vi "Disabled.vi"(7 "Robot Mode":T3, 10 "Match Info":T2={"Autonomous Elapsed Seconds"=0.0, "TeleOp Elapsed Seconds"=0.0, "Disabled Elapsed Seconds"=0.0, "Visited Autonomous"=FALSE, "Visited TeleOp"=FALSE, "Visited Disabled"=FALSE, "Autonomous Settings"={"Autonomous Style"=enum."Independent", "VI Refnum"=refnum}}, 11 "Call Context":T4) -> ()   [LabVIEW 2016]
doc: "This VI is called each time a disabled packet is received from the DS. It is often used to prepare for the next robot mode, to calibrate sensors, etc."
uses:
  <vilib>/Rock Robotics/WPI/DriverStation/WPI_DriverStationDerivedRobotMode.ctl
  <vilib>/Rock Robotics/WPI/DriverStation/WPI_DriverStationRobotMode2.ctl
  <vilib>/Rock Robotics/WPI/DriverStation/WPI_DriverStationMatch Info.ctl
  <vilib>/Rock Robotics/WPI/ThirdParty/CanMotor/TalonSRX/WPI_CANTalonSRX_GlobalStatus.ctl
  <vilib>/Rock Robotics/WPI/ThirdParty/Sensors/Pigeon IMU/CTRE_PigeonIMU_TareType.ctl
  <vilib>/Rock Robotics/WPI/ThirdParty/CanMotor/TalonSRX/WPI_CANTalonSRX_BrakeOverride.ctl
  <vilib>/Rock Robotics/WPI/Utilities/WPI_GetSetVariantRefNum.vi
  <vilib>/Rock Robotics/Network Tables/NT Read Boolean.vi
  Robot Global Data.vi
  <vilib>/Rock Robotics/Network Tables/NT Write Number.vi
  <vilib>/Rock Robotics/Network Tables/NT Write String.vi
panel:
  out "Right Drive":T1
  out "LeftDrive":T1
  out "Gear Limit Switch":bool
  out "Shooter 1":T1
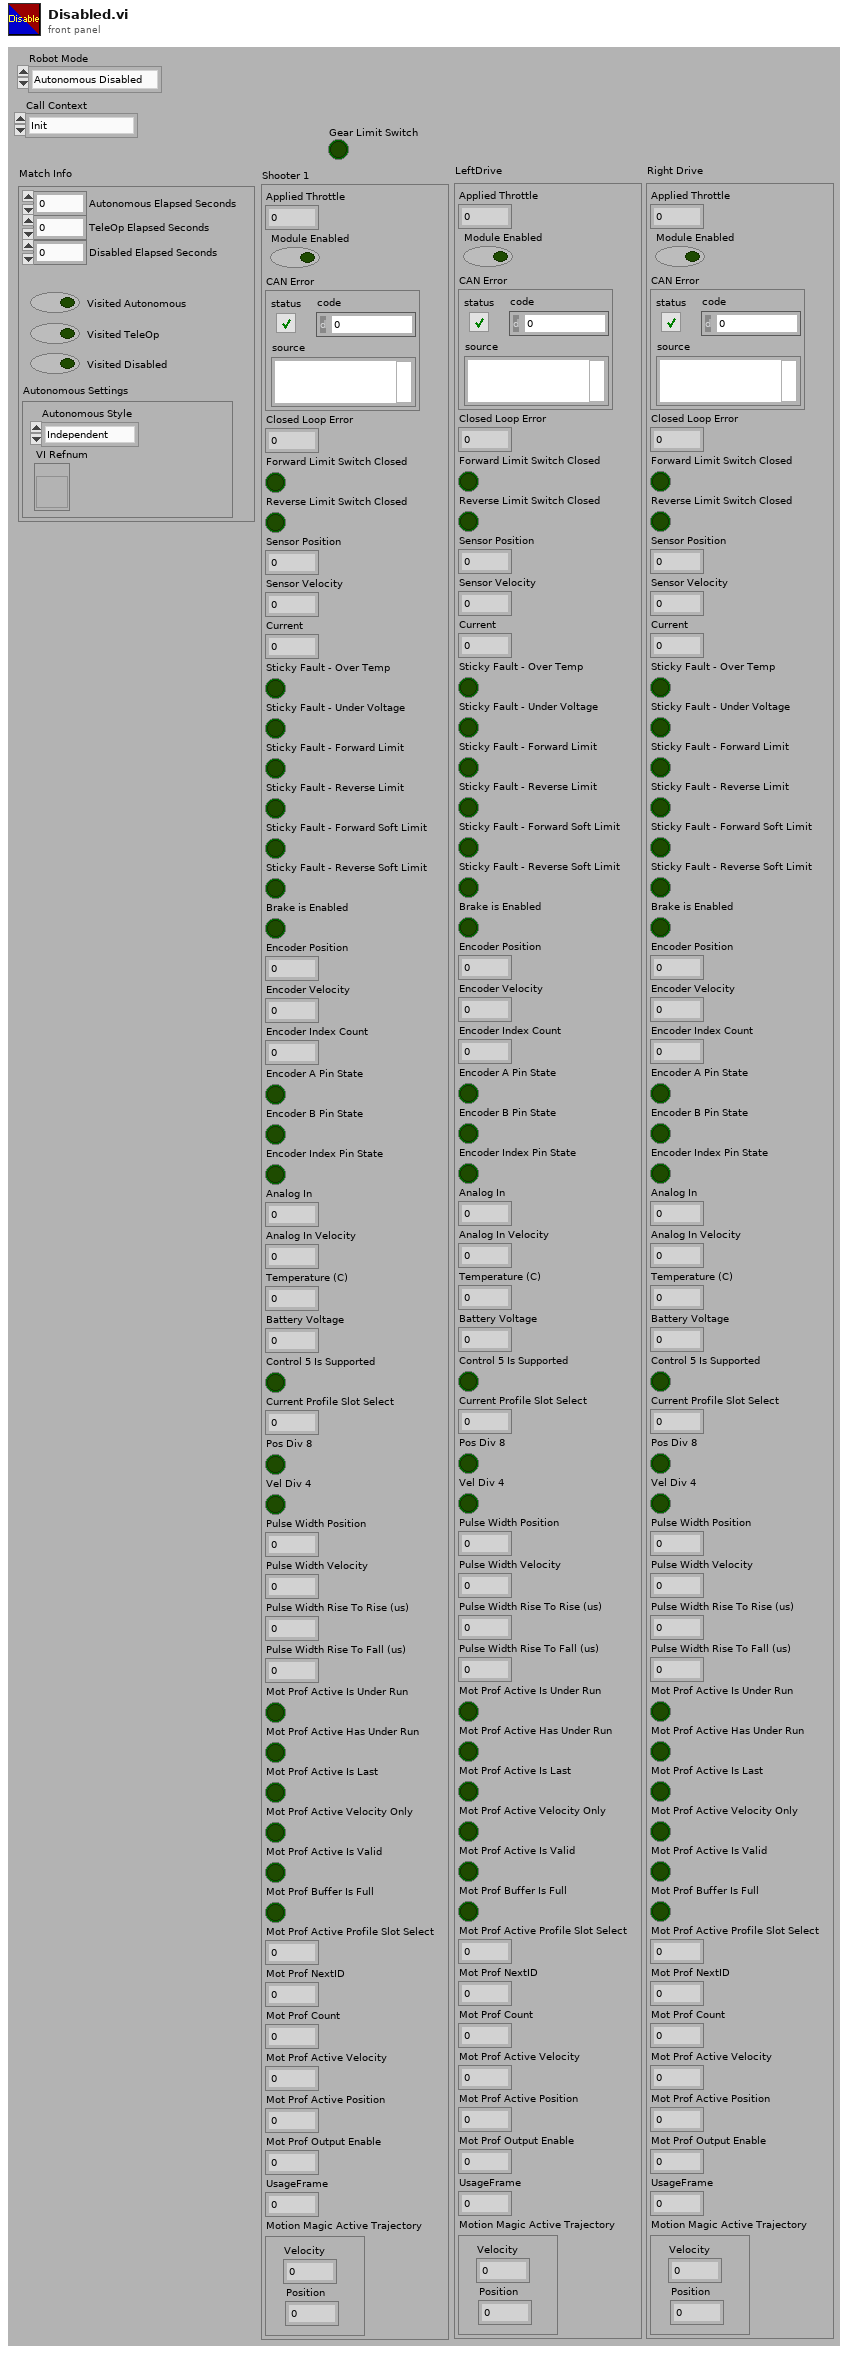
[diagram p1: front panel]
types:
  T1 = typedef "WPI_CANTalonSRX_GlobalStatus.ctl" = cluster{"Applied Throttle":dbl, "Module Enabled":bool, "CAN Error":errorcluster, "Closed Loop Error":dbl, "Forward Limit Switch Closed":bool, "Reverse Limit Switch Closed":bool, "Sensor Position":dbl, "Sensor Velocity":dbl, "Current":dbl, "Sticky Fault - Over Temp":bool, "Sticky Fault - Under Voltage":bool, "Sticky Fault - Forward Limit":bool, "Sticky Fault - Reverse Limit":bool, "Sticky Fault - Forward Soft Limit":bool, "Sticky Fault - Reverse Soft Limit":bool, "Brake is Enabled":bool, "Encoder Position":dbl, "Encoder Velocity":dbl, "Encoder Index Count":dbl, "Encoder A Pin State":bool, "Encoder B Pin State":bool, "Encoder Index Pin State":bool, "Analog In":dbl, "Analog In Velocity":dbl, "Temperature (C)":dbl, "Battery Voltage":dbl, "Control 5 Is Supported":bool, "Current Profile Slot Select":dbl, "Pos Div 8":bool, "Vel Div 4":bool, "Pulse Width Position":i32, "Pulse Width Velocity":i32, "Pulse Width Rise To Rise (us)":i32, "Pulse Width Rise To Fall (us)":i32, "Mot Prof Active Is Under Run":bool, "Mot Prof Active Has Under Run":bool, "Mot Prof Active Is Last":bool, "Mot Prof Active Velocity Only":bool, "Mot Prof Active Is Valid":bool, "Mot Prof Buffer Is Full":bool, "Mot Prof Active Profile Slot Select":i32, "Mot Prof NextID":i32, "Mot Prof Count":i32, "Mot Prof Active Velocity":dbl, "Mot Prof Active Position":dbl, "Mot Prof Output Enable":i32, "UsageFrame":u32, "Motion Magic Active Trajectory":cluster{"Velocity":dbl, "Position":dbl}}
  T2 = typedef "WPI_DriverStationMatch Info.ctl" = cluster{"Autonomous Elapsed Seconds":dbl, "TeleOp Elapsed Seconds":dbl, "Disabled Elapsed Seconds":dbl, "Visited Autonomous":bool, "Visited TeleOp":bool, "Visited Disabled":bool, "Autonomous Settings":cluster{"Autonomous Style":enum16{"Iterative", "Independent"}, "VI Refnum":refnum<vi>}}
  T3 = typedef "WPI_DriverStationRobotMode2.ctl" = enum16{"Autonomous Disabled", "Autonomous Enabled", "Teleop Disabled", "Teleop Enabled", "Disconnected", "Finish", "Test Disabled", "Test Enabled", "Emergency Stopped"}
  T4 = typedef "WPI_DriverStationDerivedRobotMode.ctl" = enum16{"Init", "Execute", "Stop"}
  T5 = typedef "WPI_CANTalonSRX_BrakeOverride.ctl" = enum8{"No Override", "Override to Coast", "Override to Brake"}
  T6 = typedef "CTRE_PigeonIMU_TareType.ctl" = u8
  T7 = typedef "WPI_MotorControlDeviceRef.ctl" = cluster{"DeviceStatus":errorcluster, "Type":T8, "PWM":cluster{"PWM Channel":T9, "DeadBand":T10}, "CAN":cluster{"Device Number":u8, "SetOutput VI Ref":variant, "GetOutput VI Ref":variant, "Enable VI Ref":variant, "Disable VI Ref":variant, "Data":variant}, "Invert":bool}
  T8 = typedef "WPI_MotorControlType.ctl" = enum16{"PWM", "CAN"}
  T9 = typedef "FPGA_DIOPWMChannel.ctl" = enum8{"PWM 0", "PWM 1", "PWM 2", "PWM 3", "PWM 4", "PWM 5", "PWM 6", "PWM 7", "PWM 8", "PWM 9", "PWM MXP 0", "PWM MXP 1", "PWM MXP 2", "PWM MXP 3", "PWM MXP 4", "PWM MXP 5", "PWM MXP 6", "PWM MXP 7", "PWM MXP 8", "PWM MXP 9", "Invalid"}
  T10 = typedef "WPI_PWMDeadband.ctl" = cluster{"Name":string, "maxPositivePwm":i32, "minPositivePwm":i32, "centerPwm":i32, "maxNegativePwm":i32, "minNegativePwm":i32, "angularRange":u16}
  T11 = typedef "WPI_DigitalInputDevRef.ctl" = cluster{"DevStatus":errorcluster, "DIO Channel":T12}
  T12 = typedef "FPGA_DIOChannel.ctl" = enum8{"DIO 0", "DIO 1", "DIO 2", "DIO 3", "DIO 4", "DIO 5", "DIO 6", "DIO 7", "DIO 8", "DIO 9", "DIO MXP 0", "DIO MXP 1", "DIO MXP 2", "DIO MXP 3", "DIO MXP 4", "DIO MXP 5", "DIO MXP 6", "DIO MXP 7", "DIO MXP 8", "DIO MXP 9", "DIO MXP 10", "DIO MXP 11", "DIO MXP 12", "DIO MXP 13", "DIO MXP 14", "DIO MXP 15", "SPI Port CS1", "SPI Port CS2", "SPI Port CS3", "SPI Port MISO", "SPI Port MOSI", "Invalid"}
  T13 = typedef "WPI_ServoDeviceRef.ctl" = cluster{"DeviceStatus":errorcluster, "PWM Channel":T9, "DeadBand":T10}
  T14 = typedef "CTRE_PigeonIMU_DeviceRef.ctl" = cluster{"DeviceStatus":errorcluster, "Device Number":u8, "Type":T15, "Device ID":u32}
  T15 = typedef "CTRE_PigeonIMU_ConnectionType.ctl" = u32
  T16 = typedef "WPI_JoystickDevRef.ctl" = cluster{"Device":T17}
  T17 = typedef "WPI_JoystickDeviceEnum.ctl" = enum16{"USB 0", "USB 1", "USB 2", "USB 3", "USB 4", "USB 5"}
  T18 = enum16{"OFF", "RED", "GREEN", "BLUE", "PURPLE", "YELLOW", "TEAL", "WHITE", "RAINBOW"}
  T19 = enum16{"SOLID", "FLASH 500ms", "FLASH 1000ms", "OFF"}
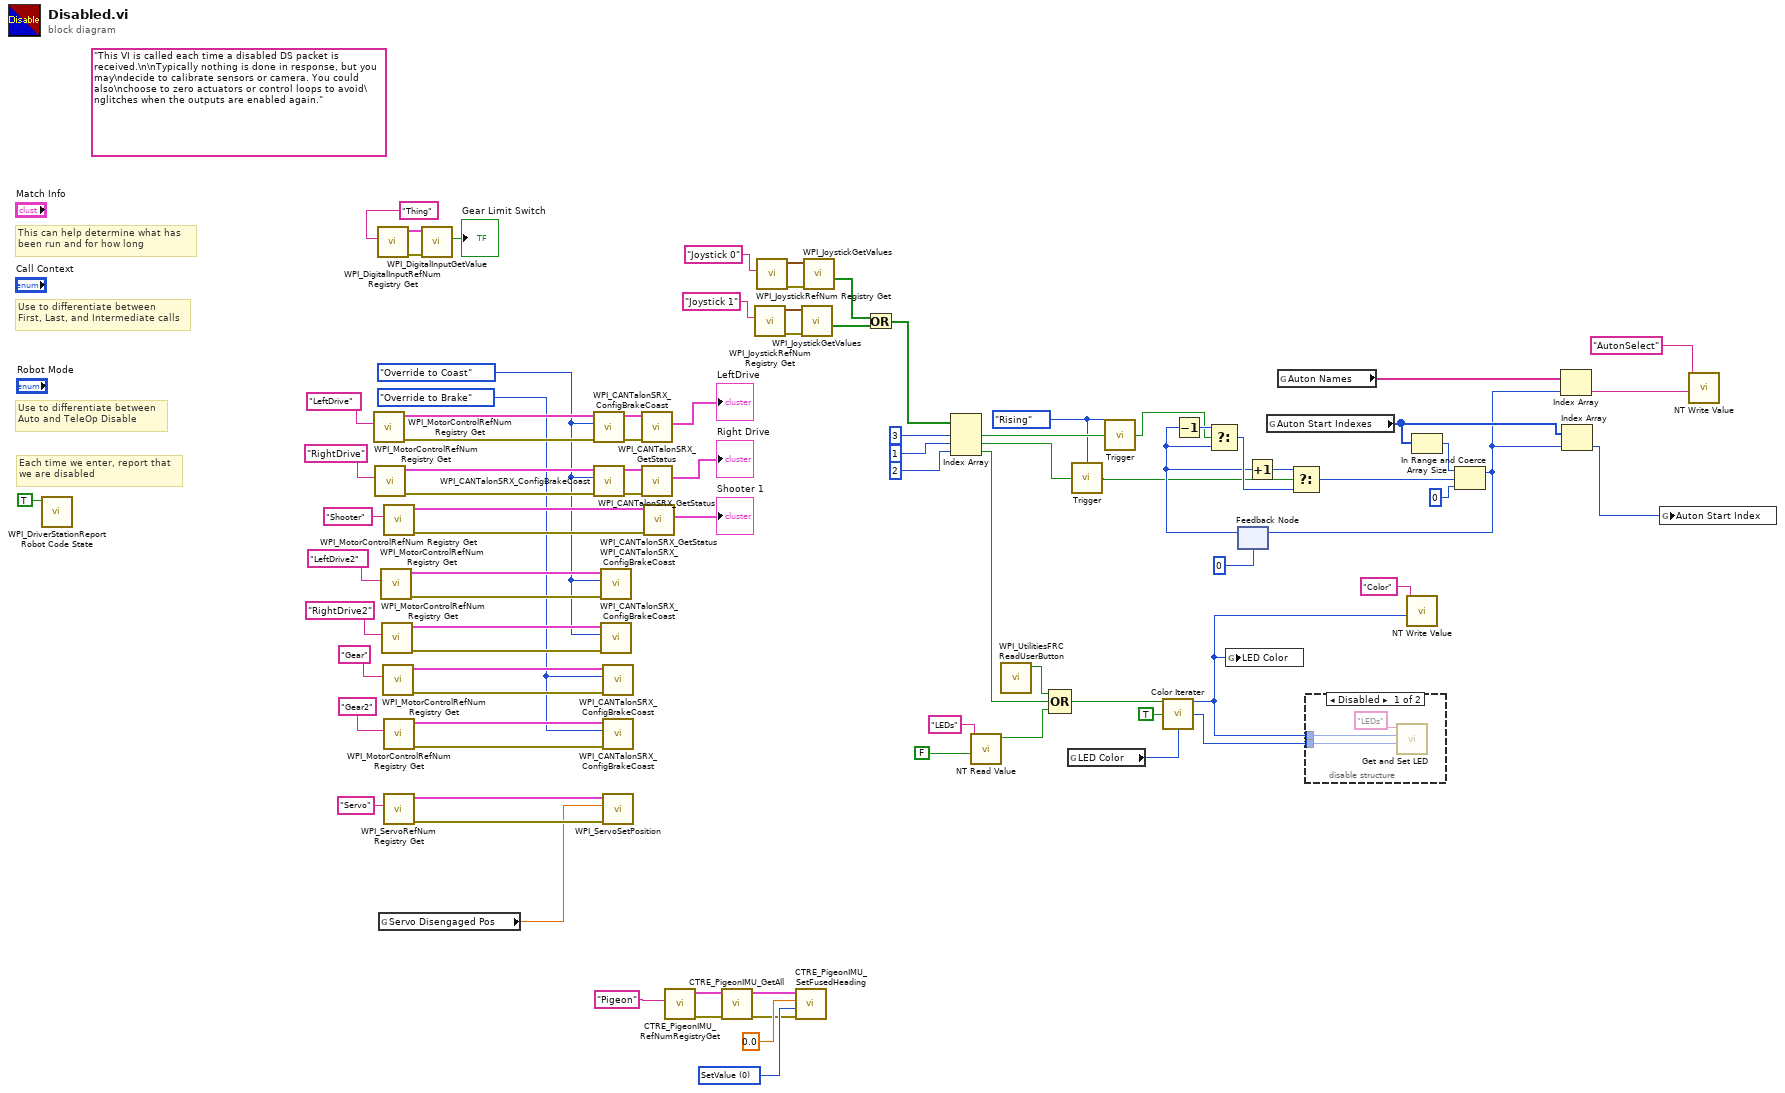
[diagram p0: block diagram]
diagram:
  w4 = WPI_CANTalonSRX_BrakeOverride."Override to Brake" ("Brake / Coast Mode")
  w27 = enum16{"Falling", "Rising", "Both"}."Rising" ("Enum")
  w51 = WPI_CANTalonSRX_BrakeOverride."Override to Coast" ("Brake / Coast Mode")
  w64 = T6 0 items=["SetValue"=0, "AddOffset"=1, "MatchCompass"=2, "SetOffset"=255] ("TareType (SetValue)")
  (unwired) "This VI is called each time a disabled DS packet is received.\n\nTypically nothing is done in response, but you may\ndecide to calibrate sensors or camera. You could also\nchoose to zero actuators or control loops to avoid\nglitches when the outputs are enabled again."
  # "Each time we enter, report that\nwe are disabled"
  # "Use to differentiate between\nFirst, Last, and Intermediate calls"
  # "This can help determine what has\nbeen run and for how long"
  # "Use to differentiate between\nAuto and TeleOp Disable"
  n1 = call <vilib>:"WPI_DriverStationReport Robot Code State.vi"("Disabled"=TRUE ("Autonomous")) -> ()  [unwired: 10 in, 1 out]
  n2 = call <vilib>:"WPI_MotorControlRefNum Registry Get.vi"("refnum name"="LeftDrive") -> ("error out"=w83:errorcluster, "MotorControlDevRef"=w85:T7)  [unwired: 9 in]
  n3 = call <vilib>:"WPI_MotorControlRefNum Registry Get.vi"("refnum name"="RightDrive") -> ("error out"=w82:errorcluster, "MotorControlDevRef"=w84:T7)  [unwired: 9 in]
  n4 = call <vilib>:"WPI_DigitalInputRefNum Registry Get.vi"("refnum name"="Thing") -> ("error out"=w75:errorcluster, "DigitalInputDevRef"=w74:T11)  [unwired: 9 in]
  n5 = global read "Robot Global Data.vi" "Servo Disengaged Pos"() -> (w1:dbl)
  n6 = call <vilib>:"WPI_MotorControlRefNum Registry Get.vi"("refnum name"="LeftDrive2") -> ("error out"=w56:errorcluster, "MotorControlDevRef"=w54:T7)  [unwired: 9 in]
  n7 = call <vilib>:"WPI_MotorControlRefNum Registry Get.vi"("refnum name"="RightDrive2") -> ("error out"=w57:errorcluster, "MotorControlDevRef"=w55:T7)  [unwired: 9 in]
  n8 = call <vilib>:"WPI_MotorControlRefNum Registry Get.vi"("refnum name"="Gear") -> ("error out"=w6:errorcluster, "MotorControlDevRef"=w8:T7)  [unwired: 9 in]
  n9 = call <vilib>:"WPI_MotorControlRefNum Registry Get.vi"("refnum name"="Shooter") -> ("error out"=w71:errorcluster, "MotorControlDevRef"=w72:T7)  [unwired: 9 in]
  n10 = call <vilib>:"WPI_MotorControlRefNum Registry Get.vi"("refnum name"="Gear2") -> ("error out"=w5:errorcluster, "MotorControlDevRef"=w7:T7)  [unwired: 9 in]
  n11 = call <vilib>:"WPI_ServoRefNum Registry Get.vi"("refnum name"="Servo") -> ("error out"=w65:errorcluster, "ServoDeviceRef"=w66:T13)  [unwired: 9 in]
  n12 = call <vilib>:"WPI_DigitalInputGetValue.vi"("error in (no error)"=w75, "DigitalInputDevRef"=w74) -> ("Value"=→"Gear Limit Switch":bool)  [unwired: 7 in, 2 out]
  n13 = call <vilib>:"WPI_CANTalonSRX_ConfigBrakeCoast.vi"("error in (no error)"=w83, "Brake / Coast Mode"=w51, "CAN Talon SRX Ref"=w85) -> ("error out"=w79:errorcluster, "CAN Talon SRX Ref"=w78:T7)  [unwired: 7 in]
  n14 = call <vilib>:"WPI_CANTalonSRX_ConfigBrakeCoast.vi"("error in (no error)"=w82, "Brake / Coast Mode"=w51, "CAN Talon SRX Ref"=w84) -> ("error out"=w81:errorcluster, "CAN Talon SRX Ref"=w80:T7)  [unwired: 7 in]
  n15 = call <vilib>:"WPI_CANTalonSRX_ConfigBrakeCoast.vi"("error in (no error)"=w56, "Brake / Coast Mode"=w51, "CAN Talon SRX Ref"=w54) -> ()  [unwired: 7 in, 2 out]
  n16 = call <vilib>:"WPI_CANTalonSRX_ConfigBrakeCoast.vi"("error in (no error)"=w57, "Brake / Coast Mode"=w51, "CAN Talon SRX Ref"=w55) -> ()  [unwired: 7 in, 2 out]
  n17 = call <vilib>:"WPI_CANTalonSRX_ConfigBrakeCoast.vi"("error in (no error)"=w6, "Brake / Coast Mode"=w4, "CAN Talon SRX Ref"=w8) -> ()  [unwired: 7 in, 2 out]
  n18 = call <vilib>:"WPI_CANTalonSRX_ConfigBrakeCoast.vi"("error in (no error)"=w5, "Brake / Coast Mode"=w4, "CAN Talon SRX Ref"=w7) -> ()  [unwired: 7 in, 2 out]
  n19 = call <vilib>:"WPI_ServoSetPosition.vi"("error in (no error)"=w65, "Position"=w1, "ServoDeviceRef"=w66) -> ()  [unwired: 7 in, 2 out]
  n20 = call <vilib>:"WPI_CANTalonSRX_GetStatus.vi"("error in (no error)"=w79, "CAN Talon SRX Ref"=w78) -> ("Talon SRX Status"=→"LeftDrive":T1)  [unwired: 7 in, 2 out]
  n21 = call <vilib>:"WPI_CANTalonSRX_GetStatus.vi"("error in (no error)"=w81, "CAN Talon SRX Ref"=w80) -> ("Talon SRX Status"=→"Right Drive":T1)  [unwired: 7 in, 2 out]
  n22 = call <vilib>:"WPI_CANTalonSRX_GetStatus.vi"("error in (no error)"=w71, "CAN Talon SRX Ref"=w72) -> ("Talon SRX Status"=→"Shooter 1":T1)  [unwired: 7 in, 2 out]
  n23 = call <vilib>:"CTRE_PigeonIMU_RefNumRegistryGet.vi"("refnum name"="Pigeon") -> ("error out"=w60:errorcluster, "PigeonIMUDevRef"=w61:T14)  [unwired: 9 in]
  n24 = call <vilib>:"CTRE_PigeonIMU_GetAll.vi"("error in (no error)"=w60, "PigeonIMUDevRef"=w61) -> ("error out"=w59:errorcluster, "PigeonIMUDevRef"=w58:T14)  [unwired: 7 in, 1 out]
  n25 = call <vilib>:"WPI_JoystickRefNum Registry Get.vi"("refnum name"="Joystick 1") -> ("error out"=w18:errorcluster, "JoystickDevRef"=w20:T16)  [unwired: 9 in]
  n26 = call <vilib>:"WPI_JoystickRefNum Registry Get.vi"("refnum name"="Joystick 0") -> ("error out"=w49:errorcluster, "JoystickDevRef"=w48:T16)  [unwired: 9 in]
  n27 = call <vilib>:"CTRE_PigeonIMU_SetFusedHeading.vi"("error in (no error)"=w59, "TareType (SetValue)"=w64, "Value"=0.0, "PigeonIMUDevRef 2"=w58) -> ()  [unwired: 6 in, 2 out]
  n28 = call <vilib>:"WPI_JoystickGetValues.vi"("error in (no error)"=w18, "JoystickDevRef"=w20) -> ("Buttons"=w16:bool[])  [unwired: 5 in, 4 out]
  n29 = call <vilib>:"WPI_JoystickGetValues.vi"("error in (no error)"=w49, "JoystickDevRef"=w48) -> ("Buttons"=w15:bool[])  [unwired: 5 in, 4 out]
  n30 = Or(x=w15, y=w16) -> (x .or. y?=w14:bool[])
  n31 = Index Array(array=w14, index #1=3 ("index"), index #2=1 ("index"), index #3=2 ("index")) -> (element #1=w30:bool, element #2=w28:bool, element #3=w21:bool)
  n32 = call-poly <vilib>:"NT Read Value.vi"("Default Value"=FALSE, "Name"="LEDs") -> ("Boolean"=w11:bool)  [unwired: 8 in, 1 out]
  n33 = call <vilib>:"WPI_UtilitiesFRC ReadUserButton.vi"() -> ("User Button"=w25:bool)  [unwired: 10 in, 1 out]
  n34 = Compound Arithmetic op=OR(w25, w21, w11) -> (w24:bool)
  n35 = global read "Robot Global Data.vi" "LED Color"() -> (w22:T18)
  n36 = call "Trigger.vi"("Enum"=w27, "Button"=w28) -> ("Trigger"=w29:bool)  [unwired: 13 in]
  n37 = call "Trigger.vi"("Enum"=w27, "Button"=w30) -> ("Trigger"=w31:bool)  [unwired: 13 in]
  n38 = call "Color Iterater.vi"("Change Color"=w24, "Disable Flash"=TRUE, "Initial Color"=w22) -> ("Color"=w2:T18, "Display Mode"=w23:T19)  [unwired: 11 in]
  n39 = global write "Robot Global Data.vi" "LED Color"(w2) -> ()
  n40 = feedback #1(0) -> (w41:i32)
  n41 = Decrement(x=w41) -> (x-1=w45:i32)
  n42 = Select(t=w45, s=w31, f=w41) -> (s? t:f=w44:i32)
  n43 = Increment(x=w41) -> (x+1=w43:i32)
  n44 = global read "Robot Global Data.vi" "Auton Start Indexes"() -> (w36:i32[])
  n45 = global read "Robot Global Data.vi" "Auton Names"() -> (w37:string[])
  n46 = Select(t=w43, s=w29, f=w44) -> (s? t:f=w40:i32)
  n47 = disable-structure shown="Disabled" {
    disable-tunnel: w23 -> [w91 _]
    disable-tunnel: w2 -> [w89 _]
    frame Disabled {
      n48 = call "Get and Set LED.vi"("Display Mode"=w91, "Color"=w89, "refnum name"="LEDs") -> ()  [unwired: 9 in]
    }
    frame Enabled {
    }
  }
  n49 = call-poly <vilib>:"NT Write Value.vi"("Numeric"=w2, "Name"="Color") -> ()  [unwired: 9 in, 1 out]
  n50 = Array Size(array=w36) -> (size(s)=w38:i32)
  n51 = In Range and Coerce(upper limit=w38, x=w40, lower limit=0) -> (coerced(x)=w35:i32)  [unwired: 1 out]
  n52 = feedback-in #1(w35) -> ()
  n53 = Index Array(array=w37, index=w35) -> (element=w33:string)
  n54 = Index Array(array=w36, index=w35) -> (element=w34:i32)
  n55 = global write "Robot Global Data.vi" "Auton Start Index"(w34) -> ()
  n56 = call-poly <vilib>:"NT Write Value.vi"("String"=w33, "Name"="AutonSelect") -> ()  [unwired: 9 in, 1 out]
